vi "Validate User Parameters.vi"(0 "destination directory":path, 5 "TLB` name":string, 7 "library":path, 11 "error in":errorcluster) -> (15 "error out":errorcluster)   [LabVIEW 2018, in "Springboard TLB`.lvlib"]
uses:
  Springboard TLB`.lvlib
  <vilib>/ErrorRing/Error Ring.xnode
  <vilib>/regexp/Match Regular Expression.xnode
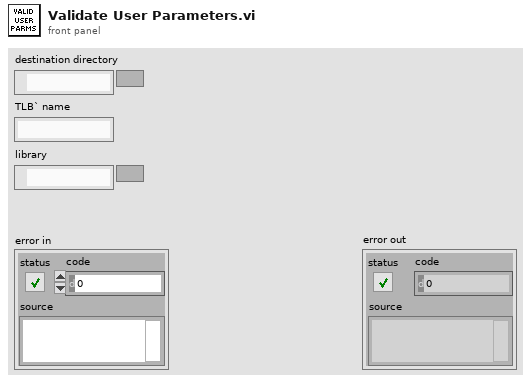
[diagram p1: front panel]
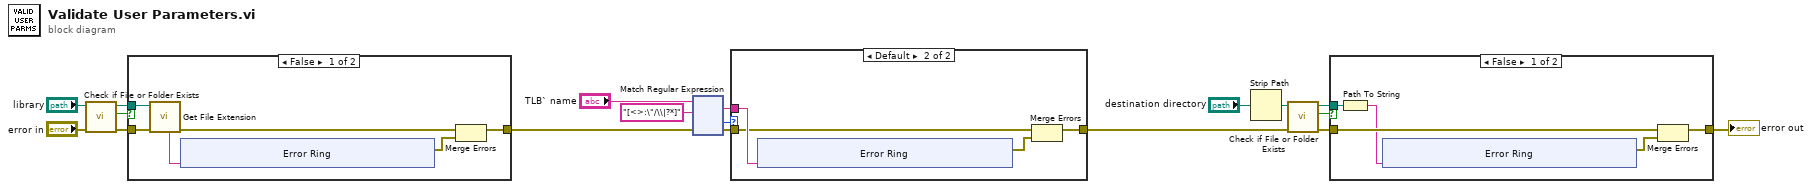
[diagram p0: block diagram]
diagram:
  n1 = call <vilib>:"Check if File or Folder Exists.vi"("error in (no error)"="error in", "path"="library") -> ("error out"=w15:errorcluster, "file or folder exists?"=w16:bool, "dup path"=w14:path)  [unwired: 7 in]
  n2 = case shown="False" w16 {
    tunnel: w15 -> [w23 w30]
    tunnel: w14 -> [w24 _]
    tunnel: [w19 w30] -> w11
    frame False {
      n3 = call <vilib>:"Get File Extension.vi"("error in (no error)"=w23, "file"=w24) -> ("error out"=w21:errorcluster, "unmodified file extension"=w22:string)  [unwired: 5 in, 3 out]
      n4 = xnode "Error Ring"("parameter 0"=w22) -> ("error out"=w20:errorcluster)
      n5 = Merge Errors(w21, w20) -> (w19:errorcluster)
    }
    frame True {
    }
  }
  n6 = xnode "Match Regular Expression"("input string"="TLB` name", "regular expression"="[<>:\"/\\|?*]", "error in"=w11) -> ("whole match"=w8:string, "offset past match"=w10:i32, "error out"=w9:errorcluster)  [unwired: 3 in, 2 out]
  n7 = case shown="Default" w10 {
    tunnel: w9 -> [w31 w34]
    tunnel: w8 -> [_ w35]
    tunnel: [w31 w32] -> w4
    frame -1 {
    }
    frame Default {
      n8 = xnode "Error Ring"("parameter 0"=w35) -> ("error out"=w33:errorcluster)
      n9 = Merge Errors(w34, w33) -> (w32:errorcluster)
    }
  }
  n10 = Strip Path(path="destination directory") -> (stripped path=w2:path)  [unwired: 1 out]
  n11 = call <vilib>:"Check if File or Folder Exists.vi"("error in (no error)"=w4, "path"=w2) -> ("error out"=w6:errorcluster, "file or folder exists?"=w7:bool, "dup path"=w5:path)  [unwired: 7 in]
  n12 = case shown="False" w7 {
    tunnel: w6 -> [w42 w51]
    tunnel: w5 -> [w43 _]
    tunnel: [w44 w51] -> w1
    frame False {
      n13 = Path To String(path=w43) -> (string=w41:string)
      n14 = xnode "Error Ring"("parameter 0"=w41) -> ("error out"=w45:errorcluster)
      n15 = Merge Errors(w42, w45) -> (w44:errorcluster)
    }
    frame True {
    }
  }
  "error out" <- w1
